vi "Stacker_Extraction_pulser_Wrapper.vi"(0 "Path":string[](array[string])=["C:\\CuspControl\\GPIB and Network\\StackerExtractionPulser.txt"], 1 "Input values":dbl[](array[numeric])=[0.0, 10.0, 0.0, 200.0]) -> ()   [LabVIEW 2018]
panel:
  out "Output enable":dbl
  out "Time (ms)":dbl
  out "Output on/off":bool
  out "Delay (ns)":dbl min=-1000000.0 max=1000000000000000.0
  out "Amplitude  (Vpp)":dbl=1.0 min=0.001 max=20.0 step=1.0 format="%#.3f"
  out "Pulse Width (ns)":dbl min=0.0 max=1000000.0 format="%.3g"
  out "error out":errorcluster
  in  "VISA resource name":refnum<visa-resource-name>="USB0::0xF4EC::0xEE38::515J19106::INSTR"
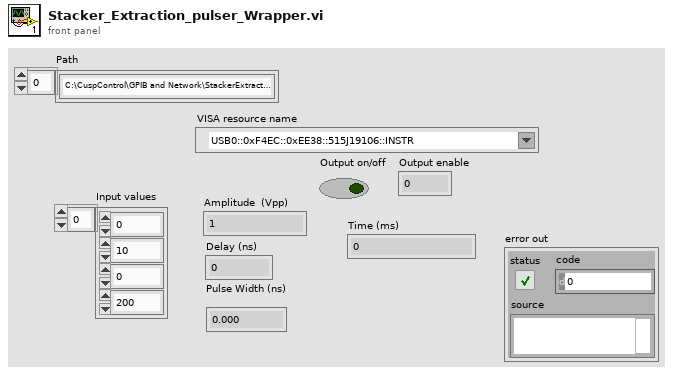
[diagram p1: front panel]
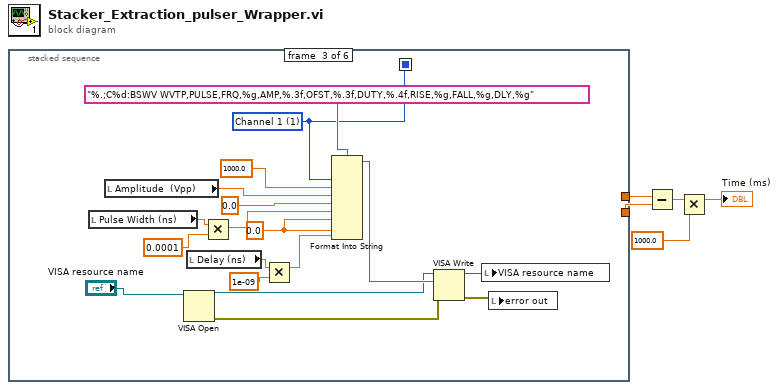
[diagram p0: block diagram]
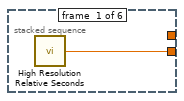
[diagram p2: hidden frame]
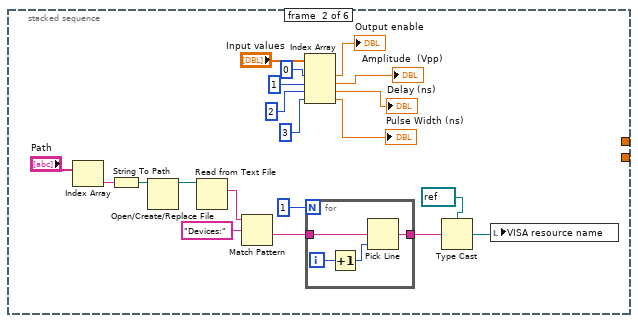
[diagram p3: hidden frame]
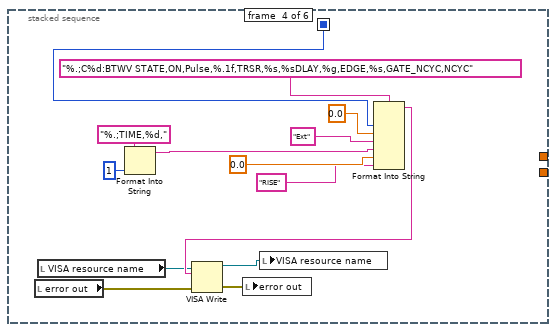
[diagram p4: hidden frame]
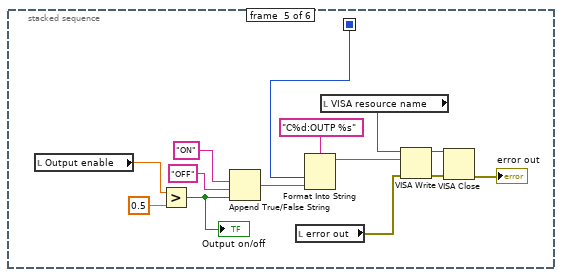
[diagram p5: hidden frame]
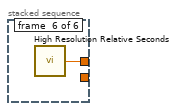
[diagram p6: hidden frame]
diagram:
  n1 = stacked-sequence {
    seq-local: [_ _ w42 _ _ _] -> [_ _ _ w49 w73 _]
    tunnel: [w6 _ _ _ _ _] -> w5
    tunnel: [_ _ _ _ _ w77] -> w1
    frame #0 {
      n2 = call <vilib>:"High Resolution Relative Seconds.vi"() -> ("relative seconds"=w6:dbl)
    }
    frame #1 {
      n3 = Index Array(array="Path") -> (element=w26:string)  [unwired: 1 in]
      n4 = String To Path(string=w26) -> (path=w20:path)
      n5 = Open/Create/Replace File(file path (use dialog)=w20) -> (refnum out=w21:refnum<file>)  [unwired: 5 in, 2 out]
      n6 = Read from Text File(file (use dialog)=w21) -> (text=w25:string)  [unwired: 3 in, 3 out]
      n7 = Match Pattern(string=w25, regular expression="Devices:") -> (after substring=w23:string)  [unwired: 1 in, 3 out]
      n8 = Index Array(array="Input values", index #1=0 ("index"), index #2=1 ("index"), index #3=2 ("index"), index #4=3 ("index")) -> (element #1=→"Output enable":dbl, element #2=→"Amplitude  (Vpp)":dbl, element #3=→"Delay (ns)":dbl, element #4=→"Pulse Width (ns)":dbl)
      n9 = for {
        N: 1 -> [_]
        tunnel: w23 -> [w28]
        tunnel: [w27] -> w18
        i -> [w30]
        n10 = Increment(x=w30) -> (x+1=w29:i32)
        n11 = Pick Line(multi-line string=w28, line index=w29) -> (output string=w27:string)  [unwired: 1 in]
      }
      n12 = Type Cast(type=refnum<visa-resource-name> refnum ("VISA resource name"), x=w18) -> (*(type *) &x=w16:refnum<visa-resource-name>)
      n13 = local write "VISA resource name"(w16) -> ()
    }
    frame #2 {
      w42 = 1 items=["Channel 1"=1, "Channel 2"=2] ("Select Channel (1:Channel 1) 2")
      w39 = 0.0 ("Rising Edge (16.8 ns) 2")
      n14 = local read "Pulse Width (ns)"() -> (w32:dbl)
      n15 = local read "Amplitude  (Vpp)"() -> (w33:dbl)
      n16 = VISA Open(VISA resource name="VISA resource name") -> (VISA resource name=w45:refnum<visa-resource-name>, error out=w44:errorcluster)  [unwired: 4 in]
      n17 = local read "Delay (ns)"() -> (w31:dbl)
      n18 = Multiply(x=w32, y=0.0001) -> (x*y=w41:dbl)
      n19 = Multiply(x=w31, y=1e-09) -> (x*y=w38:dbl)
      n20 = Format Into String(format string="%.;C%d:BSWV WVTP,PULSE,FRQ,%g,AMP,%.3f,OFST,%.3f,DUTY,%.4f,RISE,%g,FALL,%g,DLY,%g", w42, 1000.0 ("Frequency (1000 Hz)"), w33, 0.0 ("DC Offset (0.00 V)"), w41, w39, w39, w38) -> (resulting string=w47:string)  [unwired: 2 in, 1 out]
      n21 = VISA Write(VISA resource name=w45, write buffer=w47, error in (no error)=w44) -> (VISA resource name out=w35:refnum<visa-resource-name>, error out=w34:errorcluster)  [unwired: 1 out]
      n22 = local write "VISA resource name"(w35) -> ()
      n23 = local write "error out"(w34) -> ()
    }
    frame #3 {
      n24 = local read "error out"() -> (w52:errorcluster)
      n25 = local read "VISA resource name"() -> (w53:refnum<visa-resource-name>)
      n26 = Format Into String(format string="%.;TIME,%d,", 1 ("input 1")) -> (resulting string=w61:string)  [unwired: 2 in, 1 out]
      n27 = Format Into String(format string="%.;C%d:BTWV STATE,ON,Pulse,%.1f,TRSR,%s,%sDLAY,%g,EDGE,%s,GATE_NCYC,NCYC", w49, 0.0 ("Start Phase (0.0 degrees)"), "Ext" ("input 3"), w61, 0.0 ("Burst Delay (0 s)"), "RISE") -> (resulting string=w57:string)  [unwired: 2 in, 1 out]
      n28 = VISA Write(VISA resource name=w53, write buffer=w57, error in (no error)=w52) -> (VISA resource name out=w51:refnum<visa-resource-name>, error out=w50:errorcluster)  [unwired: 1 out]
      n29 = local write "error out"(w50) -> ()
      n30 = local write "VISA resource name"(w51) -> ()
    }
    frame #4 {
      n31 = local read "Output enable"() -> (w64:dbl)
      n32 = Greater?(x=w64, y=0.5) -> (0:w63:bool)
      "Output on/off" <- w63
      n33 = Append True/False String(1:w63, 2:"OFF" ("true string"), 3:"ON" ("true string")) -> (0:w68:string)  [unwired: 1 in]
      n34 = local read "error out"() -> (w70:errorcluster)
      n35 = Format Into String(format string="C%d:OUTP %s", w73, w68) -> (resulting string=w72:string)  [unwired: 2 in, 1 out]
      n36 = local read "VISA resource name"() -> (w69:refnum<visa-resource-name>)
      n37 = VISA Write(VISA resource name=w69, write buffer=w72, error in (no error)=w70) -> (VISA resource name out=w66:refnum<visa-resource-name>, error out=w65:errorcluster)  [unwired: 1 out]
      n38 = VISA Close(VISA resource name=w66, error in (no error)=w65) -> (error out=→"error out":errorcluster)
    }
    frame #5 {
      n39 = call <vilib>:"High Resolution Relative Seconds.vi"() -> ("relative seconds"=w77:dbl)
    }
  }
  n40 = Subtract(x=w1, y=w5) -> (x-y=w4:dbl)
  n41 = Multiply(x=w4, y=1000.0) -> (x*y=→"Time (ms)":dbl)
